vi "oax_gsSet Selected Item in Listbox.vi"(8 "error in (no error)":errorcluster, 9 "item name":string, 11 "control refnum":refnum<vi>) -> (0 "error out":errorcluster, 2 "actual item name":string, 3 "actual item":i32)   [LabVIEW 2017]
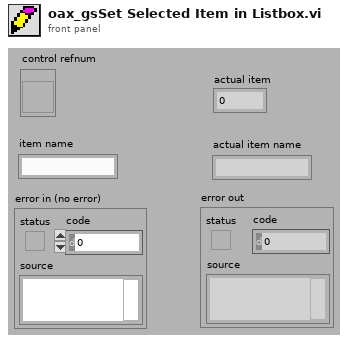
[diagram p1: front panel]
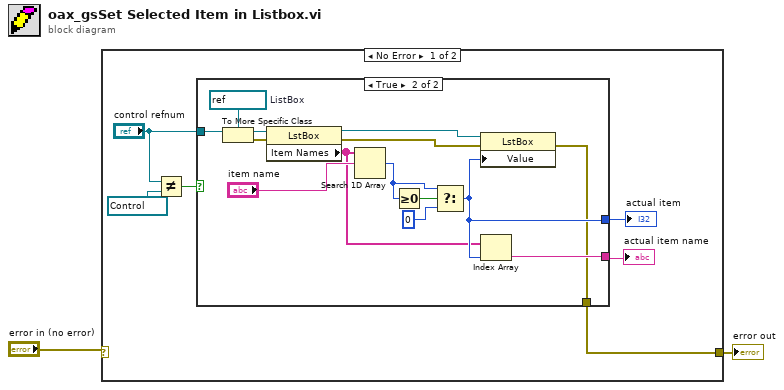
[diagram p0: block diagram]
diagram:
  n1 = case shown="No Error" "error in (no error)" {
    selector: "error in (no error)" -> [_ w23]
    tunnel: [w6 w23] -> w1
    frame No Error {
      n2 = Not Equal?(x="control refnum", y=refnum<vi> refnum) -> (x != y?=w3:bool)
      n3 = case shown="True" w3 {
        tunnel: "control refnum" -> [_ w22]
        tunnel: [_ w15] -> w8
        tunnel: [_ w13] -> w7
        tunnel: [_ w12] -> w6
        frame False {
        }
        frame True {
          w9 = refnum<vi> refnum  # ListBox
          n4 = To More Specific Class(target class=w9, reference=w22) -> (specific class reference=w19:refnum<vi>, error out=w21:errorcluster)  [unwired: 1 in]
          n5 = property class="LstBox"(reference=w19, error in=w21) -> (reference out=w10:refnum<vi>, error out=w11:errorcluster, "Item Names"=w14:string[])
          n6 = Search 1D Array(1D array=w14, element="item name") -> (index of element=w17:i32)  [unwired: 1 in]
          n7 = Greater Or Equal To 0?(x=w17) -> (x >= 0?=w18:bool)
          n8 = Select(t=w17, s=w18, f=0) -> (s? t:f=w15:i32)
          n9 = property class="LstBox"(reference=w10, error in=w11, "Value"=w15) -> (error out=w12:errorcluster)  [unwired: 1 out]
          n10 = Index Array(array=w14, index=w15) -> (element=w13:string)
        }
      }
      "actual item name" <- w7
      "actual item" <- w8
    }
    frame Error {
    }
  }
  "error out" <- w1
